vi "Add Channels.vi"(8 "error in":errorcluster, 10 "Channel in":refnum<class "Channel.lvclass">[](array[class]), 11 "Node Ptr in":T1 format="%.0x") -> (0 "error out":errorcluster, 3 "Node Ptr out":T1 format="%.0x")   [LabVIEW 2024, in "FPGA Addon System Explorer.lvlib"]
uses:
  FPGA Addon System Explorer.lvlib
  <vilib>/NI VeriStand/Custom Device API/Custom Device Item Ref.ctl
  Parser/Channel/Channel.lvclass
  <vilib>/NI VeriStand/Custom Device API/Custom Device Channel.ctl
  <vilib>/NI VeriStand/Custom Device API/Custom Device Channel Type.ctl
  <vilib>/NI VeriStand/Custom Device API/Custom Device API.lvlib
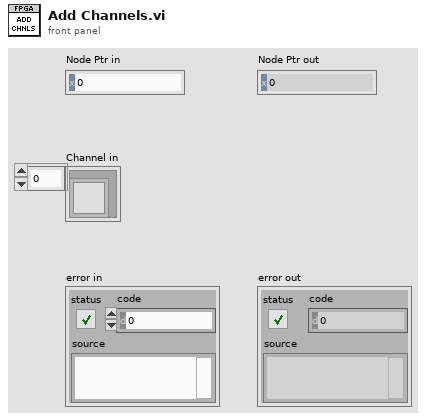
[diagram p1: front panel]
types:
  T1 = typedef "Custom Device API.lvlib/Custom Device Item Ref.ctl" = u64
  T2 = typedef "Custom Device API.lvlib/Custom Device Channel.ctl" = cluster{"Type":T3, "Units":string, "Default Value":dbl, "Faultable":bool, "Scalable":bool}
  T3 = typedef "Custom Device API.lvlib/Custom Device Channel Type.ctl" = enum16{"Input", "Output"}
  T4 = cluster{"Name":string, "Type":enum16{"Input", "Output"}, "TypeGUID":string, "Identifier":string, "DefaultValue":dbl, "Errors":cluster{"Key":string, "IsError":bool, "Code":u32, "Message":string}[], "Description":string, "RowDim":i32, "ColDim":i32, "Units":string, "Scalability":bool, "Faultability":bool}
  T5 = cluster{"Key":string, "IsError":bool, "Code":u32, "Message":string}[]
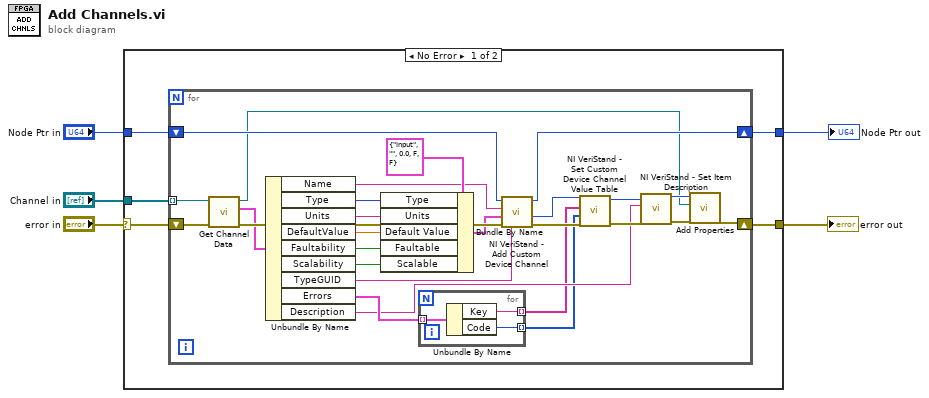
[diagram p0: block diagram]
diagram:
  n1 = case shown="No Error" "error in" {
    selector: "error in" -> [w9 w42]
    tunnel: [w10 w42] -> w5
    tunnel: "Node Ptr in" -> [w8 w41]
    tunnel: [w7 w41] -> w2
    tunnel: "Channel in" -> [w6 _]
    frame No Error {
      n2 = for {
        tunnel: w6 -> [w21] mode=indexing
        shift-right: [w32] -> w10
        shift-left: w9 -> [w37]
        shift-right: [w17] -> w7
        shift-left: w8 -> [w18]
        n3 = call "Get Channel Data.vi"("error in"=w37, "Channel in"=w21) -> ("error out"=w36:errorcluster, "Channel Data"=w31:T4, "Channel out"=w11:refnum<class "Channel.lvclass">)  [unwired: 7 in]
        n4 = Unbundle By Name(w31) -> ("Name"=w23:string, "Type"=w30:enum16{"Input", "Output"}, "Units"=w29:string, "DefaultValue"=w28:dbl, "Faultability"=w27:bool, "Scalability"=w26:bool, "TypeGUID"=w22:string, "Errors"=w20:T5, "Description"=w19:string)
        n5 = Bundle By Name(cluster=T2 {"Type"=enum."Input", "Units"="", "Default Value"=0.0, "Faultable"=FALSE, "Scalable"=FALSE} ("Channel"), "Type"=w30, "Units"=w29, "Default Value"=w28, "Faultable"=w27, "Scalable"=w26) -> (w24:T2)
        n6 = for {
          tunnel: w20 -> [w40] mode=indexing
          tunnel: [w39] -> w15 mode=indexing
          tunnel: [w38] -> w14 mode=indexing
          n7 = Unbundle By Name(w40) -> ("Key"=w39:string, "Code"=w38:u32)
        }
        n8 = call <vilib>:"NI VeriStand - Add Custom Device Channel.vi"("GUID (Default Channel)"=w22, "error in (no error)"=w36, "Channel"=w24, "Channel Name"=w23, "Parent Ref in"=w18) -> ("error out"=w34:errorcluster, "Channel Ref"=w13:T1, "Parent Ref out"=w17:T1)  [unwired: 3 in, 1 out]
        n9 = call <vilib>:"NI VeriStand - Set Custom Device Channel Value Table.vi"("error in (no error)"=w34, "Values"=w14, "Names"=w15, "Channel Ref in"=w13) -> ("error out"=w35:errorcluster, "Channel Ref out"=w16:T1)  [unwired: 6 in]
        n10 = call <vilib>:"NI VeriStand - Set Item Description.vi"("error in (no error)"=w35, "Description"=w19, "Item Ref in"=w16) -> ("error out"=w33:errorcluster, "Item Ref out"=w12:T1)  [unwired: 6 in, 1 out]
        n11 = call "Add Properties.vi"("error in"=w33, "Item in"=w11, "Node Ptr in"=w12) -> ("error out"=w32:errorcluster)  [unwired: 7 in, 1 out]
      }
    }
    frame Error {
    }
  }
  "error out" <- w5
  "Node Ptr out" <- w2
